vi "Get Node-ID.vi"(11 "CANopen Message in":refnum<class "CANopen Message.lvclass">) -> (2 "Node-ID":u8, 3 "CANopen Message out":refnum<class "CANopen Message.lvclass">)   [LabVIEW 2024, in "CANopen Master.lvlib" / "CANopen Message.lvclass"]
uses:
  CANopen Message.lvclass
  CANopen Message.lvclass/CANopen Message.ctl
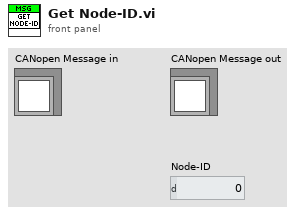
[diagram p1: front panel]
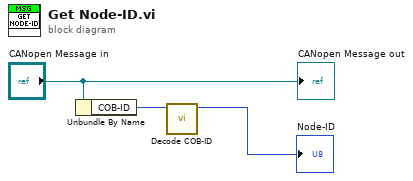
[diagram p0: block diagram]
diagram:
  n1 = Unbundle By Name("CANopen Message in") -> ("COB-ID"=w2:u32)
  n2 = call "Decode COB-ID.vi"("COD-ID"=w2) -> ("Node-ID"=→"Node-ID":u8)  [unwired: 9 in, 1 out]
  "CANopen Message out" <- "CANopen Message in"
